vi "单步流程命令.vi"(7 "是否启用通讯通知":bool, 8 "error in (no error)":errorcluster, 10 "流程控制":T2, 11 "Slave ID":T1) -> (0 "error out":errorcluster)   [LabVIEW 2016, in "质控单元V1.lvlib"]
uses:
  <vilib>/Plasmionique/MB Master/MB_Master/MB_Master.lvclass
  <vilib>/Plasmionique/MB Master/MB Master.lvlib
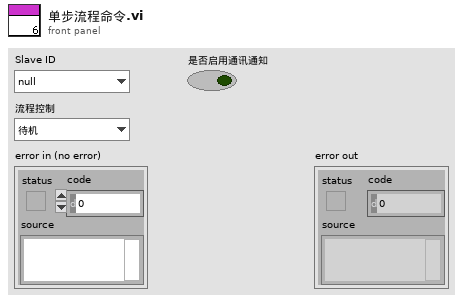
[diagram p1: front panel]
types:
  T1 = typedef "质控单元V1.lvlib/质控slave id.ctl" = enum16{"null", "氨氮", "总磷", "CODMn", "CODCr", "总氮"}
  T2 = typedef "质控单元V1.lvlib/质控流程控制.ctl" = enum16{"待机", "润洗", "进样", "加标", "排液", "搅拌"}
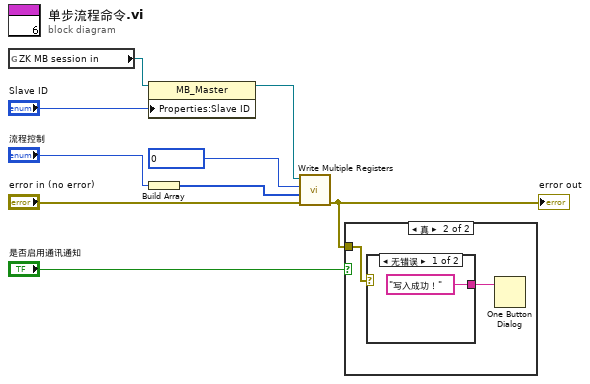
[diagram p0: block diagram]
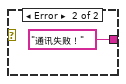
[diagram p3: hidden frame]
diagram:
  n1 = global read "ZK非断电保存全局变量.vi" "ZK MB session in"() -> (w8:refnum<class "MB_Master.lvclass">)
  n2 = property class="MB_Master"(reference=w8, "Properties:Slave ID"="Slave ID") -> (reference out=w6:refnum<class "MB_Master.lvclass">)  [unwired: 1 in, 1 out]
  n3 = Build Array("流程控制") -> (w4:T2[])
  n4 = call <vilib>:"Write Multiple Registers.vi"("error in (no error)"="error in (no error)", "values"=w4, "starting address"=u16 0, "MB session in"=w6) -> ("error out"=w2:errorcluster)  [unwired: 6 in, 1 out]
  "error out" <- w2
  n5 = case shown="真" "是否启用通讯通知" {
    tunnel: w2 -> [_ w11]
    frame False {
    }
    frame True {
      n6 = case shown="无错误" w11 {
        tunnel: ["写入成功！" "通讯失败！"] -> w10
        frame No Error {
        }
        frame Error {
        }
      }
      n7 = One Button Dialog(message=w10) -> ()  [unwired: 1 in, 1 out]
    }
  }
